vi "Select a Bliley Switcher2023.vi"(2 "Bliley Relay Box":u8, 3 "Bliley Relay Box 2":u8, 4 "Oscillator Under Test":u16) -> (0 "GPIB Address":u8, 1 "RF Position":u8)   [LabVIEW 2023]
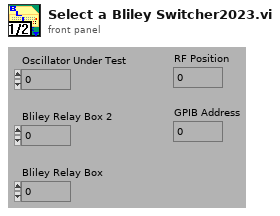
[diagram p1: front panel]
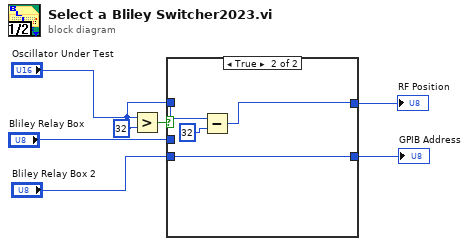
[diagram p0: block diagram]
diagram:
  n1 = Greater?(x="Oscillator Under Test", y=u16 32) -> (0:w2:bool)
  n2 = case shown="True" w2 {
    tunnel: "Bliley Relay Box 2" -> [_ w13]
    tunnel: "Bliley Relay Box" -> [w9 _]
    tunnel: [w9 w13] -> w5
    tunnel: [w8 w11] -> w6
    tunnel: "Oscillator Under Test" -> [w8 w12]
    frame False {
    }
    frame True {
      n3 = Subtract(x=w12, y=u16 32) -> (x-y=w11:u16)
    }
  }
  "RF Position" <- w6
  "GPIB Address" <- w5
